vi "Cryostation.getAll.vi"(8 "error in (no error)":errorcluster, 11 "instrument.Cryostation in":refnum<class "instrument.Cryostation.lvclass">) -> (0 "error out":errorcluster, 2 "getAll":T1, 3 "instrument.Cryostation out":refnum<class "instrument.Cryostation.lvclass">)   [LabVIEW 2019, in "instrument.Cryostation.lvclass"]
uses:
  instrument.Cryostation.lvclass
  Typedefs/Cryostation.getAll--cluster.ctl
  instrument.Cryostation.lvclass/instrument.Cryostation.ctl
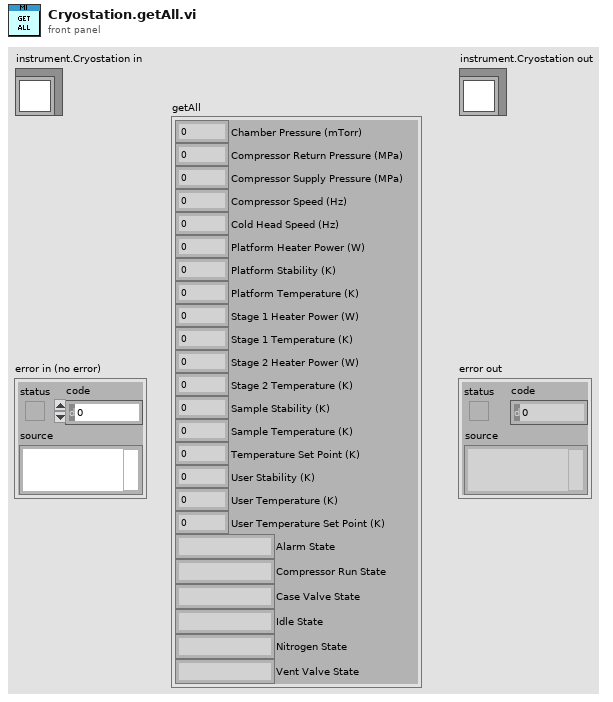
[diagram p1: front panel]
types:
  T1 = typedef "instrument.Cryostation.lvclass/Cryostation.getAll--cluster.ctl" = cluster{"Chamber Pressure (mTorr)":dbl, "Compressor Return Pressure (MPa)":dbl, "Compressor Supply Pressure (MPa)":dbl, "Compressor Speed (Hz)":dbl, "Cold Head Speed (Hz)":dbl, "Platform Heater Power (W)":dbl, "Platform Stability (K)":dbl, "Platform Temperature (K)":dbl, "Stage 1 Heater Power (W)":dbl, "Stage 1 Temperature (K)":dbl, "Stage 2 Heater Power (W)":dbl, "Stage 2 Temperature (K)":dbl, "Sample Stability (K)":dbl, "Sample Temperature (K)":dbl, "Temperature Set Point (K)":dbl, "User Stability (K)":dbl, "User Temperature (K)":dbl, "User Temperature Set Point (K)":dbl, "Alarm State":string, "Compressor Run State":string, "Case Valve State":string, "Idle State":string, "Nitrogen State":string, "Vent Valve State":string}
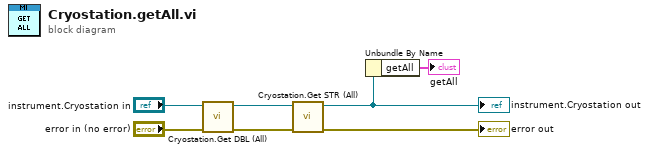
[diagram p0: block diagram]
diagram:
  n1 = call "Cryostation.Get DBL (All).vi"("error in (no error)"="error in (no error)", "instrument.Cryostation in"="instrument.Cryostation in") -> ("error out"=w2:errorcluster, "instrument.Cryostation out"=w3:refnum<class "instrument.Cryostation.lvclass">)  [unwired: 8 in]
  n2 = call "Cryostation.Get STR (All).vi"("error in (no error)"=w2, "instrument.Cryostation in"=w3) -> ("error out"=→"error out":errorcluster, "instrument.Cryostation out"=w4:refnum<class "instrument.Cryostation.lvclass">)  [unwired: 8 in]
  "instrument.Cryostation out" <- w4
  n3 = Unbundle By Name(w4) -> ("getAll"=→"getAll":T1)
